vi "XLP80_EA_Globals.vi"() -> ()   [LabVIEW 2021]
uses:
  XLP80_EA_TDefsCluster_EA Feedback.ctl
  XLP80_EA_TDefsCluster_EA Setpoint.ctl
  XLP80_EA_TDefsCluster_EA Setpoint_Reku.ctl
panel:
  in  "Setpoint EA Rekuperation":T1 {"Set Power" min=0 max=60000 step=100 format="%.0f W"; "Set Voltage" min=0 max=90 step=1 format="%.2f V"; "Set Current" min=0 max=840 step=1 format="%.2f A"}
  out "Error EA Stack":bool
  out "Feedback EA Stack":T2 {"Voltage" format="%.2f V"; "Current" format="%.2f A"}
  in  "Setpoint EA Stack":T3 {"Set Voltage" min=0 max=90 step=1 format="%.2f V"; "Set Current" min=0 max=210 step=1 format="%.2f A"}
  out "Error EA Batterie":bool
  out "Feedback EA Batterie":T2 {"Voltage" format="%.2f V"; "Current" format="%.2f A"}
  in  "Setpoint EA Batterie":T3 {"Set Voltage" min=0 max=90 step=1 format="%.2f V"; "Set Current" min=0 max=210 step=1 format="%.2f A"}
  out "Error EA Rekuperation":bool
  out "Feedback EA Rekuperation":T2 {"Voltage" format="%.2f V"; "Current" format="%.2f A"}
  # "Set EA Load"
  # "Feedback EA Load"
  # "Set EA Load"
  # "Feedback EA Load"
  # "Set EA Load"
  # "Feedback EA Load"
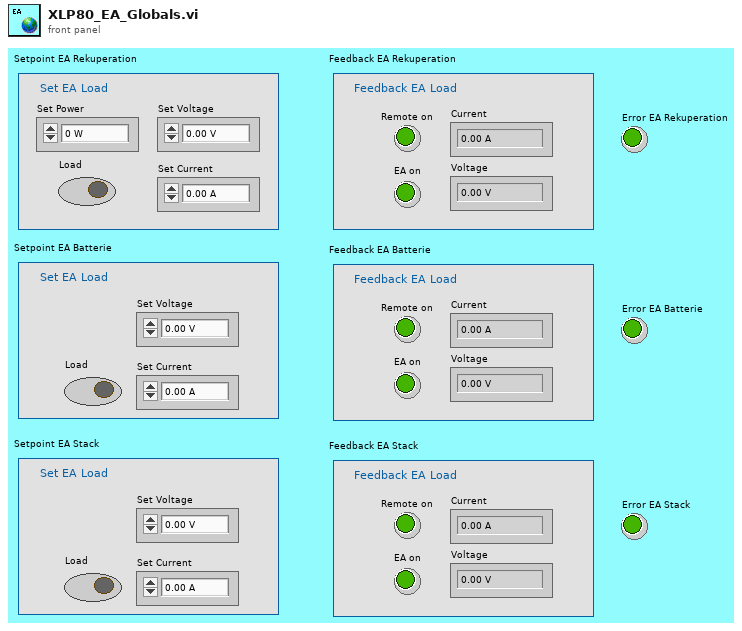
[diagram p1: front panel]
types:
  T1 = typedef "XLP80_EA_TDefsCluster_EA Setpoint_Reku.ctl" = cluster{"Load":bool, "Set Current":sgl, "Set Voltage":sgl, "Set Power":sgl}
  T2 = typedef "XLP80_EA_TDefsCluster_EA Feedback.ctl" = cluster{"EA on":bool, "Current":sgl, "Voltage":sgl, "Remote on":bool}
  T3 = typedef "XLP80_EA_TDefsCluster_EA Setpoint.ctl" = cluster{"Load":bool, "Set Current":sgl, "Set Voltage":sgl}
diagram:
